vi "IsSessionLoaded.vi"(8 "error in (no error)":errorcluster, 11 "session id in":i32) -> (0 "error out":errorcluster, 2 "SessionLoaded":bool, 3 "session id out":i32)   [LabVIEW 2018, in "libonnx_wrapper.lvlib"]
doc: "/**\n * @brief Проверить, загружена ли сессия в память\n * \n * Функция возвращает текущий статус сессии. Полезно для проверки перед вызовом\n * инференса, особенно если использовалась функция UnloadSession.\n * \n * @param sessionId [IN] ID сессии, полученный от CreateSession\n * \n * @return int32: 1 если сессия активна и модель загружена в память\n * @return int32: 0 если сессия не найдена или выгружена из памяти\n */\nint IsSessionLoaded(int sessionId);"
uses:
  libonnx_wrapper.lvlib
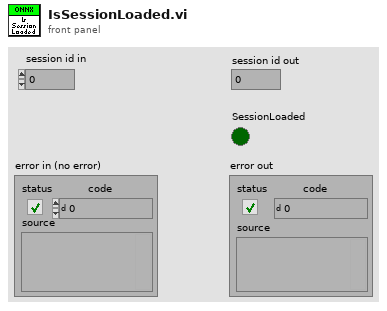
[diagram p1: front panel]
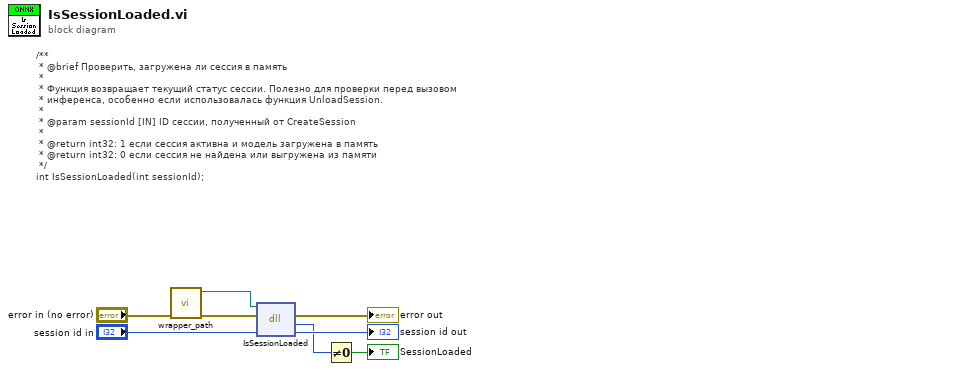
[diagram p0: block diagram]
diagram:
  # "/**\n * @brief Проверить, загружена ли сессия в память\n * \n * Функция возвращает текущий статус сессии. Полезно для проверки перед вызовом\n * инференса, особенно если использовалась функция UnloadSession.\n * \n * @param sessionId [IN] ID сессии, полученный от CreateSession\n * \n * @return int32: 1 если сессия активна и модель загружена в память\n * @return int32: 0 если сессия не найдена или выгружена из памяти\n */\nint IsSessionLoaded(int sessionId);"
  n1 = call "wrapper_path.vi"("error in (no error)"="error in (no error)") -> ("error out"=w6:errorcluster, "wrapper path"=w5:path)  [unwired: 9 in]
  n2 = dll-call lib="home/ivan/LabVIEWData/ONNX/Test/libonnx_wrapper/unix64/libonnx_wrapper.so" fn="IsSessionLoaded"(path in=w5, error in=w6, "sessionId"="session id in") -> (error out=→"error out":errorcluster, "IsSessionLoaded"=w2:i32, "sessionId"=→"session id out":i32)  [unwired: 1 in, 1 out]
  n3 = Not Equal To 0?(x=w2) -> (x != 0?=→"SessionLoaded":bool)
